vi "PWM2 Set Duty Cycle.vi"(9 "DutyCycle":u16, 10 "ChannelIndex":u8, 11 "DevHandle":i32) -> (3 "function return":i32)   [LabVIEW 2010, in "usb2pwm.lvlib"]
doc: "int WINAPI PWM2_SetDutyCycle(int DevHandle, unsigned char ChannelIndex, unsigned short DutyCycle);"
uses:
  usb2pwm.lvlib
  USB2XXX/trunk/USB2XXX/USB2XXX/vs2019/Release/USB2XXX.dll
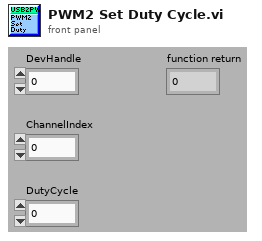
[diagram p1: front panel]
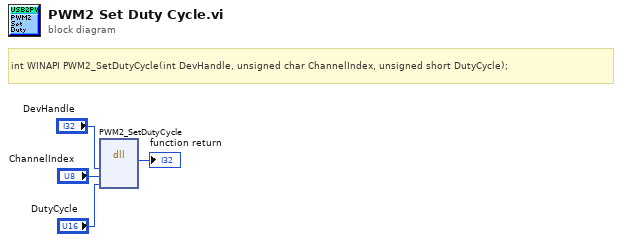
[diagram p0: block diagram]
diagram:
  # "int WINAPI PWM2_SetDutyCycle(int DevHandle, unsigned char ChannelIndex, unsigned short DutyCycle);"
  n1 = dll-call lib="E:/Projects/USB2XXX/trunk/USB2XXX/USB2XXX/vs2019/Release/USB2XXX.*" fn="PWM2_SetDutyCycle"("DevHandle"="DevHandle", "ChannelIndex"="ChannelIndex", "DutyCycle"="DutyCycle") -> (→"function return":i32)  [unwired: 6 in, 2 out]
